vi "Read_Temperature.vi"(8 "error in (no error)":errorcluster, 11 "Omega CN9600 series.lvclass":refnum<class "Omega CN9600 series.lvclass">) -> (0 "error out":errorcluster, 2 "Temperature":dbl, 3 "Omega CN9600 series.lvclass 2":refnum<class "Omega CN9600 series.lvclass">)   [LabVIEW 2014, in "Omega CN9600 series.lvclass"]
uses:
  Omega CN9600 series.lvclass
  Omega CN9600 series.lvclass/Omega CN9600 series.ctl
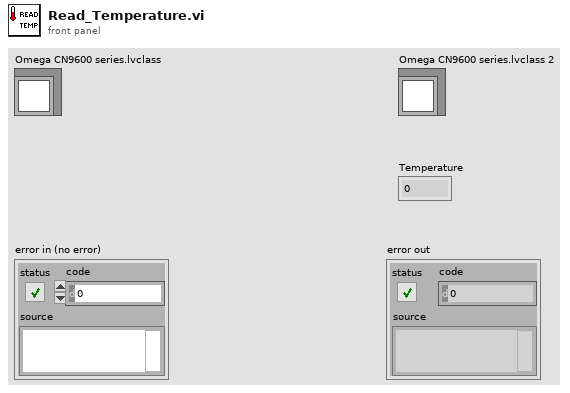
[diagram p1: front panel]
types:
  T1 = typedef "Omega CN9600 series.lvclass/Serial_Config_Omega.ctl" = cluster{"Baud":u32, "Flow Ctl":u16, "Parity":u16, "COM Port":refnum<visa-resource-name>, "Address":u8}
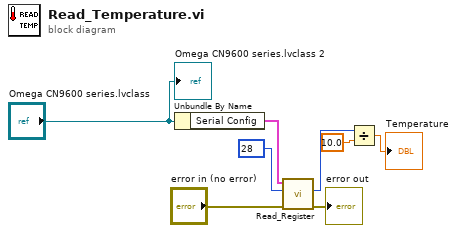
[diagram p0: block diagram]
diagram:
  n1 = Unbundle By Name("Omega CN9600 series.lvclass") -> ("Serial Config"=w8:T1)
  n2 = call "Read_Register.vi"("error in (no error)"="error in (no error)", "Address"=u16 28, "Serial Config"=w8) -> ("error out"=→"error out":errorcluster, "Value"=w6:u16)  [unwired: 6 in, 1 out]
  n3 = Divide(x=w6, y=10.0) -> (x/y=→"Temperature":dbl)
  "Omega CN9600 series.lvclass 2" <- "Omega CN9600 series.lvclass"
